vi "Main.vi"() -> ()   [LabVIEW 2012]
uses:
  file_action_enum.ctl
  <vilib>/Utility/file.llb/Read From Spreadsheet File (string).vi
  <vilib>/Utility/file.llb/Write To Spreadsheet File (string).vi
panel:
  out "counter 2":i32
  in  "choice":T1=enum."convert 16-bit tiff"
  out "Slide":dbl(slide) scale=0.0..1.0
  out "counter":i32
  out "filesmoved log path":path
  out "file to transfer":path
  out "error out 2":errorcluster
  out "error out":errorcluster
  in  "button:start":bool
  in  "button:stop":bool
  in  "Tab Control":enum32{"Main", "Debug"}(tab)
  in  "Source direcory":path
  in  "Destination directory":path
  in  "file age (sec.)":dbl
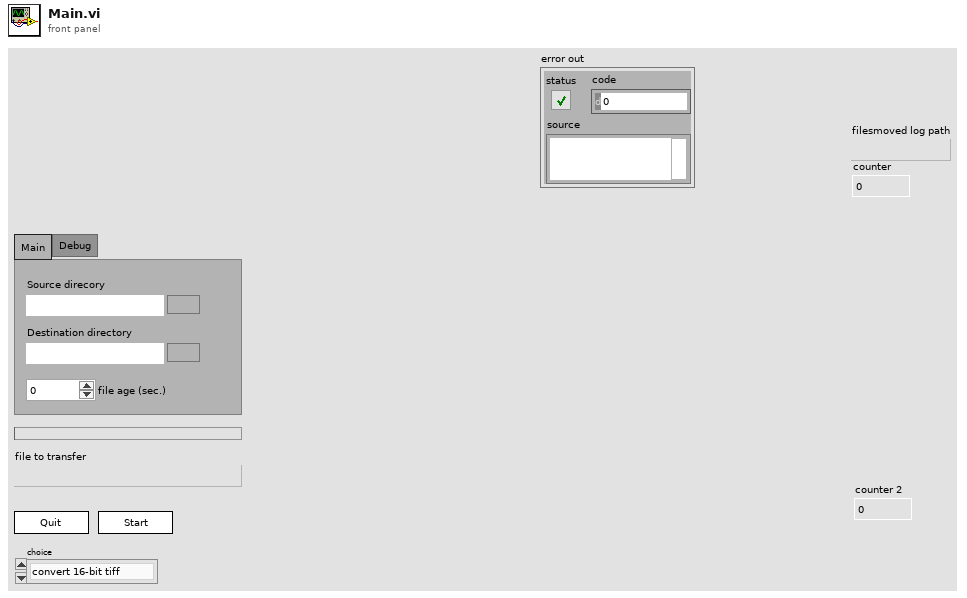
[diagram p1: front panel]
types:
  T1 = typedef "file_action_enum.ctl" = enum16{"move", "convert 16-bit tiff", "convert 8-bit tiff"}
  T2 = enum16{"open", "replace", "create", "open or create", "replace or create", "replace or create with confirmation"}
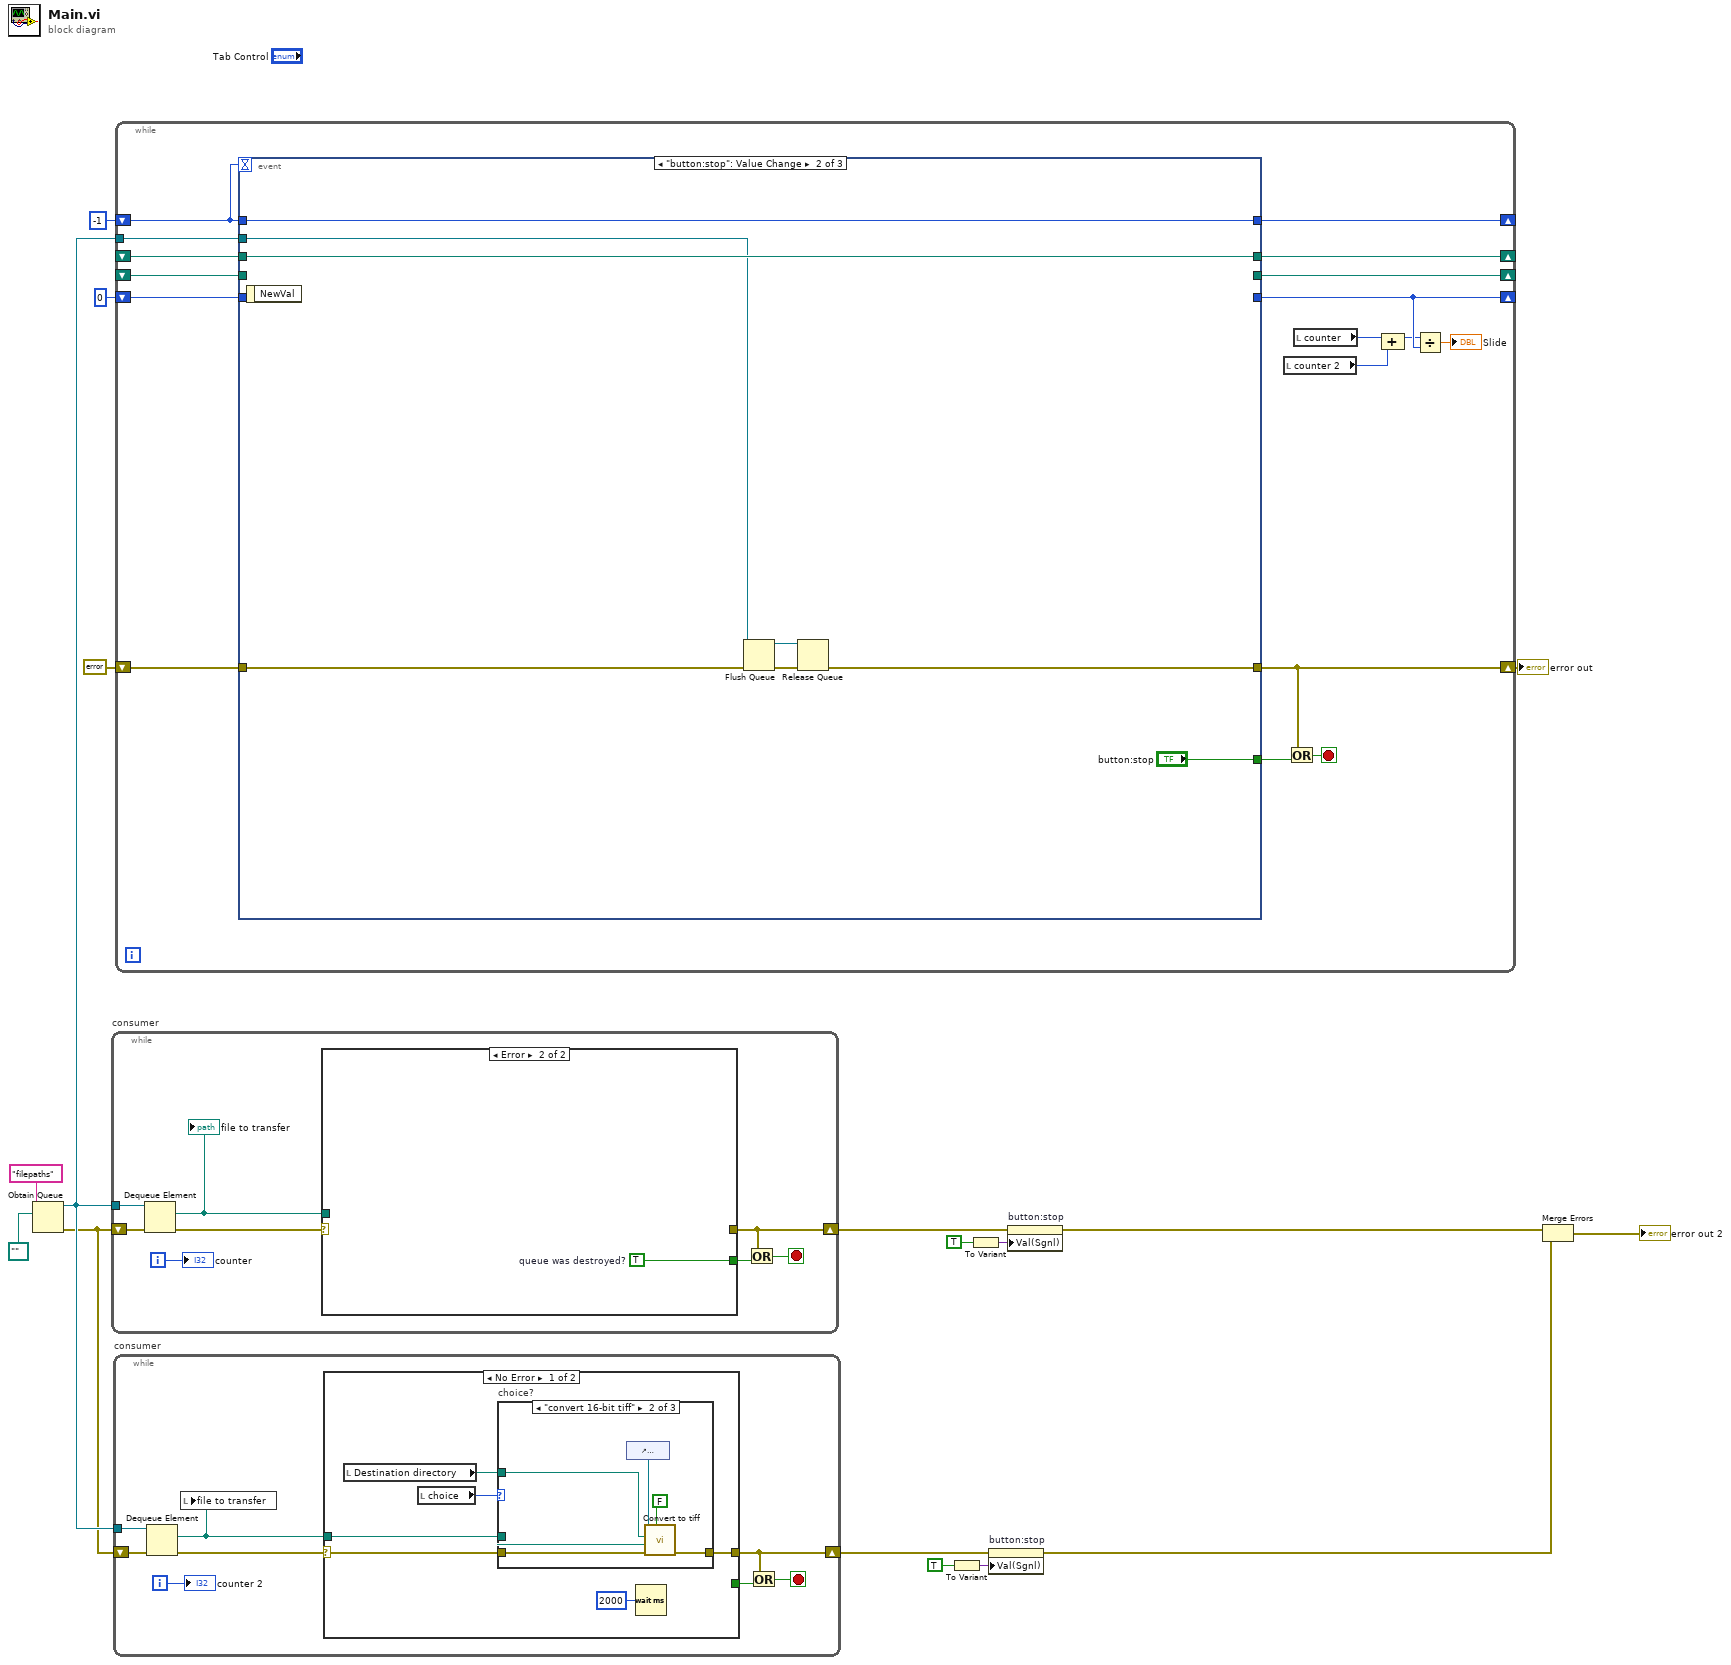
[diagram p0: block diagram]
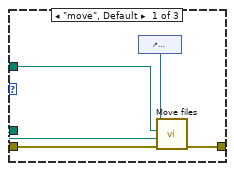
[diagram p2: hidden frame]
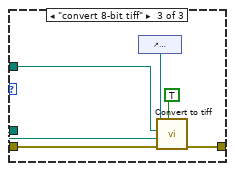
[diagram p3: hidden frame]
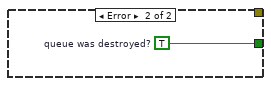
[diagram p4: hidden frame]
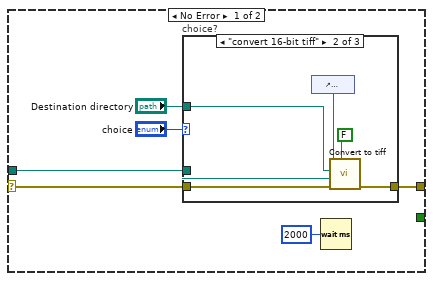
[diagram p5: hidden frame]
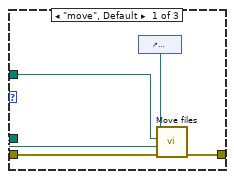
[diagram p6: hidden frame]
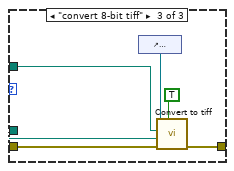
[diagram p7: hidden frame]
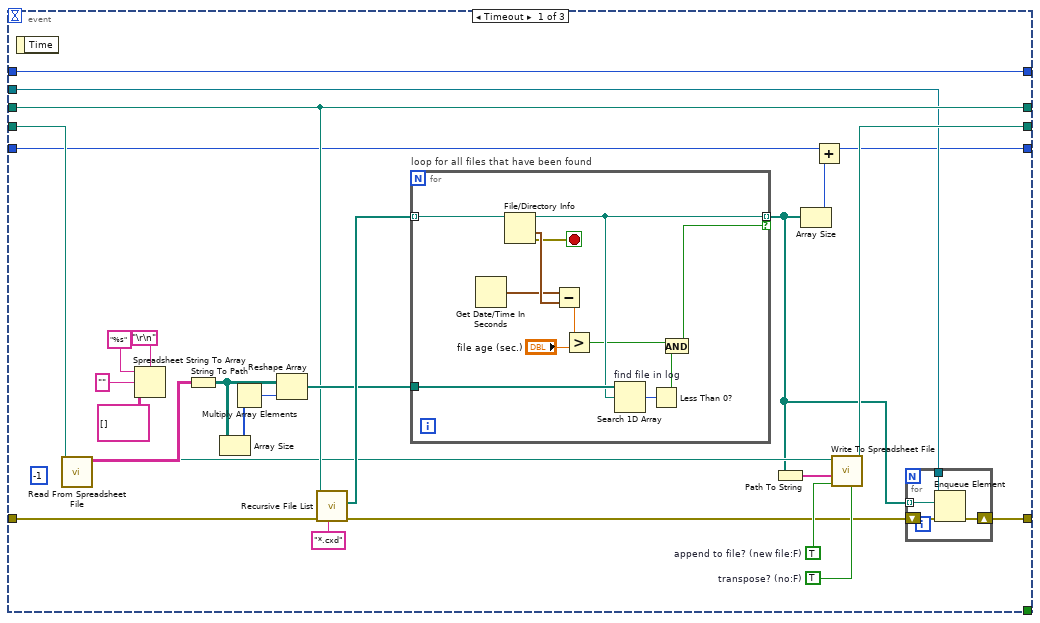
[diagram p8: hidden frame]
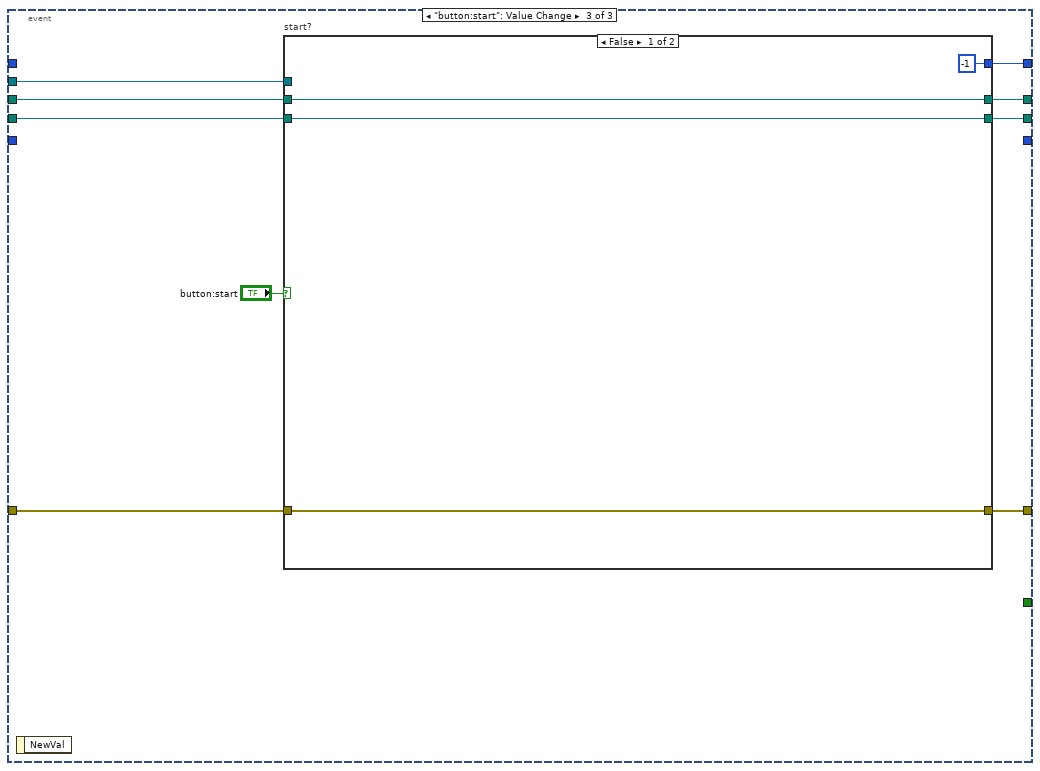
[diagram p9: hidden frame]
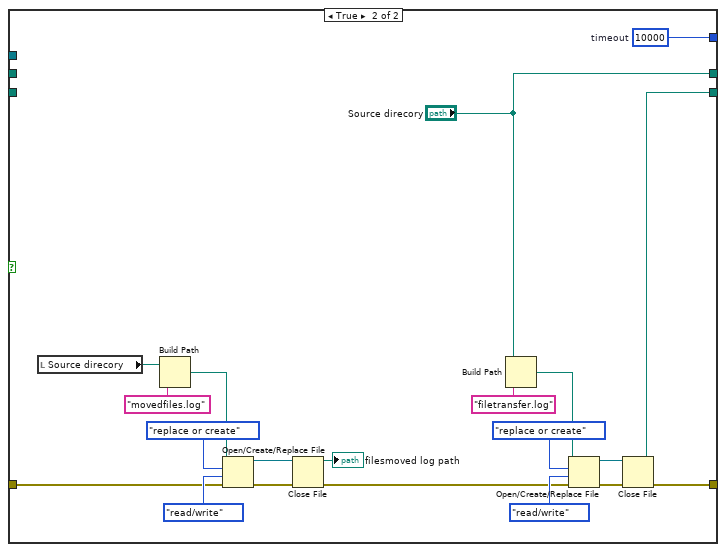
[diagram p10: hidden frame]
diagram:
  n1 = Obtain Queue(name (unnamed)="filepaths", element data type=path "" ("Destination directory")) -> (queue out=w8:refnum<queue>, error out=w7:errorcluster)  [unwired: 3 in, 1 out]
  n2 = while "consumer" {
    tunnel: w8 -> [w25]
    shift-right: [w19] -> w12
    shift-left: w7 -> [w24]
    i -> [w18]
    stop <- w20 stop-if-true
    n3 = Dequeue Element(queue=w25, error in (no error)=w24) -> (element=w23:path, error out=w22:errorcluster)  [unwired: 1 in, 2 out]
    "file to transfer" <- w23
    n4 = case shown="Error" w22 {
      selector: w22 -> [w30 _]
      tunnel: w23 -> [w31 _]
      tunnel: [w29 _] -> w19
      tunnel: [_ w49] -> w21
      frame No Error {
        n5 = case "choice?" shown="\"convert 16-bit tiff\"" "choice" {
          tunnel: w31 -> [w36 w42 w48]
          tunnel: w30 -> [w35 w41 w47]
          tunnel: [w34 w40 w46] -> w29
          tunnel: "Destination directory" -> [w33 w39 w45]
          frame "move", Default {
            n6 = control-ref of="filesmoved log path"() -> (w32:refnum<vi>)
            n7 = call "Move files.vi"("error in (no error)"=w35, "source file"=w36, "Destination directory"=w33, "Path in"=w32) -> ("error out"=w34:errorcluster)  [unwired: 7 in]
          }
          frame "convert 16-bit tiff" {
            n8 = control-ref of="filesmoved log path"() -> (w38:refnum<vi>)
            n9 = call "Convert to tiff.vi"("downcast to 8-bit? (F)"=FALSE, "error in (no error)"=w41, "source file"=w42, "Destination directory"=w39, "reference to path"=w38) -> ("error out"=w40:errorcluster)  [unwired: 6 in]
          }
          frame "convert 8-bit tiff" {
            n10 = control-ref of="filesmoved log path"() -> (w44:refnum<vi>)
            n11 = call "Convert to tiff.vi"("downcast to 8-bit? (F)"=TRUE, "error in (no error)"=w47, "source file"=w48, "Destination directory"=w45, "reference to path"=w44) -> ("error out"=w46:errorcluster)  [unwired: 6 in]
          }
        }
        n12 = Wait (ms)(milliseconds to wait=u32 2000) -> ()  [unwired: 1 out]
      }
      frame Error {
        w49 = TRUE  # queue was destroyed?
      }
    }
    n13 = Or(x=w19, y=w21) -> (x .or. y?=w20:bool)
    "counter" <- w18
  }
  n14 = while "consumer" {
    tunnel: w8 -> [w57]
    shift-right: [w52] -> w4
    shift-left: w7 -> [w56]
    i -> [w51]
    stop <- w53 stop-if-true
    n15 = Dequeue Element(queue=w57, error in (no error)=w56) -> (element=w50:path, error out=w55:errorcluster)  [unwired: 1 in, 2 out]
    n16 = local write "file to transfer"(w50) -> ()
    n17 = case shown="No Error" w55 {
      selector: w55 -> [w62 _]
      tunnel: w50 -> [w63 _]
      tunnel: [w61 _] -> w52
      tunnel: [_ w81] -> w54
      frame No Error {
        n18 = local read "Destination directory"() -> (w58:path)
        n19 = local read "choice"() -> (w59:T1)
        n20 = case "choice?" shown="\"convert 16-bit tiff\"" w59 {
          tunnel: w63 -> [w68 w74 w80]
          tunnel: w62 -> [w67 w73 w79]
          tunnel: [w66 w72 w78] -> w61
          tunnel: w58 -> [w65 w71 w77]
          frame "move", Default {
            n21 = control-ref of="filesmoved log path"() -> (w64:refnum<vi>)
            n22 = call "Move files.vi"("error in (no error)"=w67, "source file"=w68, "Destination directory"=w65, "Path in"=w64) -> ("error out"=w66:errorcluster)  [unwired: 7 in]
          }
          frame "convert 16-bit tiff" {
            n23 = control-ref of="filesmoved log path"() -> (w70:refnum<vi>)
            n24 = call "Convert to tiff.vi"("downcast to 8-bit? (F)"=FALSE, "error in (no error)"=w73, "source file"=w74, "Destination directory"=w71, "reference to path"=w70) -> ("error out"=w72:errorcluster)  [unwired: 6 in]
          }
          frame "convert 8-bit tiff" {
            n25 = control-ref of="filesmoved log path"() -> (w76:refnum<vi>)
            n26 = call "Convert to tiff.vi"("downcast to 8-bit? (F)"=TRUE, "error in (no error)"=w79, "source file"=w80, "Destination directory"=w77, "reference to path"=w76) -> ("error out"=w78:errorcluster)  [unwired: 6 in]
          }
        }
        n27 = Wait (ms)(milliseconds to wait=u32 2000) -> ()  [unwired: 1 out]
      }
      frame Error {
        w81 = TRUE  # queue was destroyed?
      }
    }
    n28 = Or(x=w52, y=w54) -> (x .or. y?=w53:bool)
    "counter 2" <- w51
  }
  n29 = while {
    shift-right: [w97] -> _
    shift-left: -1 -> [w96]
    shift-right: [w95] -> _
    shift-left: _ -> [w98]
    shift-right: [w91] -> w15
    shift-left: errorcluster {"status"=FALSE, "code"=0, "source"=""} ("error out") -> [w94]
    shift-right: [w93] -> _
    shift-left: _ -> [w92]
    tunnel: w8 -> [w88]
    shift-right: [w86] -> _
    shift-left: 0 -> [w87]
    stop <- w90 stop-if-true
    n30 = event shown="[1] \"button:stop\": Value Change" {
      selector: _ -> [_ _ _]
      dyn-events: _ -> [_ _ _]
      timeout: w96 -> [_ _ _]
      tunnel: w98 -> [w118 _ w151]
      tunnel: [_ "button:stop" _] -> w89
      tunnel: [w106 w148 w158] -> w97
      tunnel: w96 -> [w106 w148 _]
      tunnel: [w110 _ w156] -> w95
      tunnel: [w103 w142 w155] -> w91
      tunnel: w94 -> [w112 w143 w154]
      tunnel: [w120 w147 w157] -> w93
      tunnel: w92 -> [w120 w147 w152]
      tunnel: w88 -> [w105 w146 w150]
      tunnel: [w100 _ _] -> w86
      tunnel: w87 -> [w99 _ _]
      event Timeout {
        w107 = TRUE  # transpose? (no:F)
        w108 = TRUE  # append to file? (new file:F)
        (unwired) -1 ("count")
        n31 = event-data() -> ()  [unwired: 1 in, 1 out]
        n32 = call-poly <vilib>:"Read From Spreadsheet File.vi"("file path (dialog if empty)"=w118) -> ("all rows"=w114:string[][], "new file path (Not A Path if cancelled)"=w111:path)  [unwired: 6 in, 3 out]
        n33 = Spreadsheet String To Array(delimiter (Tab)="\r\n", format string="%s", spreadsheet string="", array type (2D Dbl)=string[][] []) -> ()  [unwired: 1 out]
        n34 = String To Path(string=w114) -> (path=w123:path[][])
        n35 = Array Size(array=w123) -> (size(s)=w117:i32[])
        n36 = Multiply Array Elements(1:w117) -> (0:w116:i32)
        n37 = Reshape Array(w123, w116) -> (w122:path[])
        n38 = call <vilib>:"Recursive File List.vi"("pattern"="*.cxd", "error in (no error)"=w112, "Folder Path"=w120) -> ("error out"=w104:errorcluster, "All Files in Dir"=w125:path[])  [unwired: 4 in, 3 out]
        n39 = for "loop for all files that have been found" {
          tunnel: w125 -> [w141] mode=indexing
          tunnel: [w135] -> w102 mode=indexing if=w131
          tunnel: w122 -> [w136]
          stop <- w137 stop-if-true
          n40 = Get Date/Time In Seconds() -> (seconds since 1Jan1904=w139:timestamp)
          n41 = File/Directory Info(path=w141) -> (path out=w135:path, last mod=w140:timestamp, error out=w137:errorcluster)  [unwired: 1 in, 4 out]
          n42 = Subtract(x=w139, y=w140) -> (x-y=w130:dbl)
          n43 = Greater?(x=w130, y="file age (sec.)") -> (0:w133:bool)
          n44 = Search 1D Array "find file in log"(1D array=w136, element=w135) -> (index of element=w134:i32)  [unwired: 1 in]
          n45 = Less Than 0?(x=w134) -> (x < 0?=w132:bool)
          n46 = And(x=w133, y=w132) -> (x .and. y?=w131:bool)
        }
        n47 = Path To String(path=w102) -> (string=w109:string[])
        n48 = Array Size(array=w102) -> (size(s)=w101:i32)
        n49 = Add(x=w99, y=w101) -> (x+y=w100:i32)
        n50 = call-poly <vilib>:"Write To Spreadsheet File.vi"("transpose? (no:F)"=w107, "append to file? (new file:F)"=w108, "1D data"=w109, "file path (dialog if empty)"=w111) -> ("new file path (Not A Path if cancelled)"=w110:path)  [unwired: 4 in]
        n51 = for {
          tunnel: w105 -> [w129]
          tunnel: w102 -> [w126] mode=indexing
          shift-right: [w127] -> w103
          shift-left: w104 -> [w128]
          n52 = Enqueue Element(queue=w129, element=w126, error in (no error)=w128) -> (error out=w127:errorcluster)  [unwired: 1 in, 2 out]
        }
      }
      event "button:stop": Value Change {
        n53 = event-data() -> ()  [unwired: 1 in, 1 out]
        n54 = Flush Queue(queue=w146, error in (no error)=w143) -> (queue out=w145:refnum<queue>, error out=w144:errorcluster)  [unwired: 1 out]
        n55 = Release Queue(queue=w145, error in (no error)=w144) -> (error out=w142:errorcluster)  [unwired: 1 in, 2 out]
      }
      event "button:start": Value Change {
        n56 = event-data() -> ()  [unwired: 1 in, 1 out]
        n57 = case "start?" shown="False" "button:start" {
          tunnel: [-1 ("timeout") w182] -> w158
          tunnel: [w161 "Source direcory"] -> w157
          tunnel: [w160 w175] -> w156
          tunnel: [w159 w173] -> w155
          tunnel: w154 -> [w159 w164]
          tunnel: w152 -> [w161 _]
          tunnel: w151 -> [w160 _]
          tunnel: w150 -> [_ _]
          frame False {
          }
          frame True {
            w182 = 10000  # timeout
            n58 = local read "Source direcory"() -> (w172:path)
            n59 = Build Path(base path=w172, name or relative path="movedfiles.log") -> (appended path=w171:path)
            n60 = Open/Create/Replace File(file path (use dialog)=w171, error in=w164, operation (0:open)=T2."replace or create", access (0:read/write)=enum16{"read/write", "read-only", "write-only"}."read/write") -> (refnum out=w167:refnum<file>, error out=w165:errorcluster)  [unwired: 2 in, 1 out]
            n61 = Close File(refnum=w167, error in=w165) -> (path=→"filesmoved log path":path, error out=w163:errorcluster)
            n62 = Build Path(base path="Source direcory", name or relative path="filetransfer.log") -> (appended path=w181:path)
            n63 = Open/Create/Replace File(file path (use dialog)=w181, error in=w163, operation (0:open)=T2."replace or create", access (0:read/write)=enum16{"read/write", "read-only", "write-only"}."read/write") -> (refnum out=w176:refnum<file>, error out=w174:errorcluster)  [unwired: 2 in, 1 out]
            n64 = Close File(refnum=w176, error in=w174) -> (path=w175:path, error out=w173:errorcluster)
          }
        }
      }
    }
    n65 = local read "counter 2"() -> (w84:i32)
    n66 = Or(x=w91, y=w89) -> (x .or. y?=w90:bool)
    n67 = local read "counter"() -> (w83:i32)
    n68 = Compound Arithmetic op=ADD(w83, w84) -> (w82:i32)
    n69 = Divide(x=w82, y=w86) -> (x/y=→"Slide":dbl)
  }
  "error out" <- w15
  n70 = To Variant(anything=TRUE) -> (Variant=w6:variant)
  n71 = To Variant(anything=TRUE) -> (Variant=w10:variant)
  n72 = property on="button:stop" class="Bool"(error in=w4, "Val(Sgnl)"=w6) -> (error out=w3:errorcluster)  [unwired: 1 in, 1 out]
  n73 = property on="button:stop" class="Bool"(error in=w12, "Val(Sgnl)"=w10) -> (error out=w2:errorcluster)  [unwired: 1 in, 1 out]
  n74 = Merge Errors(w2, w3) -> (→"error out 2":errorcluster)
